vi "update.vi"(8 "error in (no error)":errorcluster, 11 "ScanHeadMH100729FPGA in":refnum<class "ScanHeadMH100729FPGA.lvclass">) -> (0 "error out":errorcluster, 3 "ScanHeadMH100729FPGA out":refnum<class "ScanHeadMH100729FPGA.lvclass">)   [LabVIEW 2010, in "ScanHeadMH100729FPGA.lvclass"]
uses:
  ScanHeadMH100729FPGA.lvclass
  Trajectory/GenericTrajectory/GenericTrajectory/GenericTrajectory.lvclass
  Trajectory/TrajectoryMG100122GenericFPGA/TrajectoryMG100122GenericFPGA/TrajectoryMG100122GenericFPGA.lvclass
  ScanHeadMH100729FPGA.lvclass/ScanHeadMH100729FPGA.ctl
  AnalogOut/GenericAnalogOut/GenericAnalogOut/GenericAnalogOut.lvclass
  common/classes/SpaceVector/SpaceVector/SpaceVector.lvclass
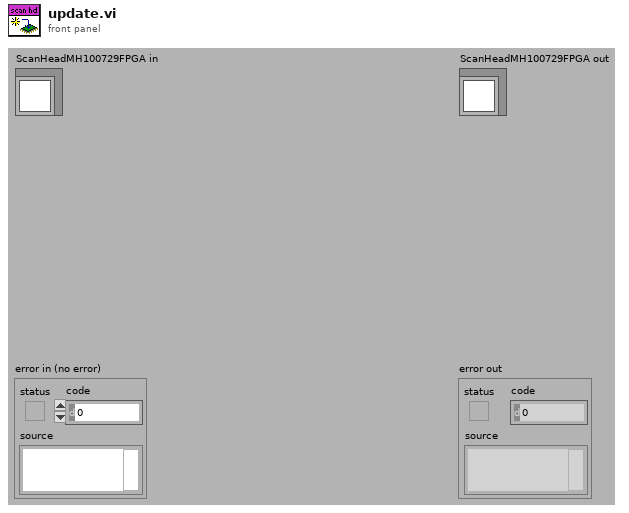
[diagram p1: front panel]
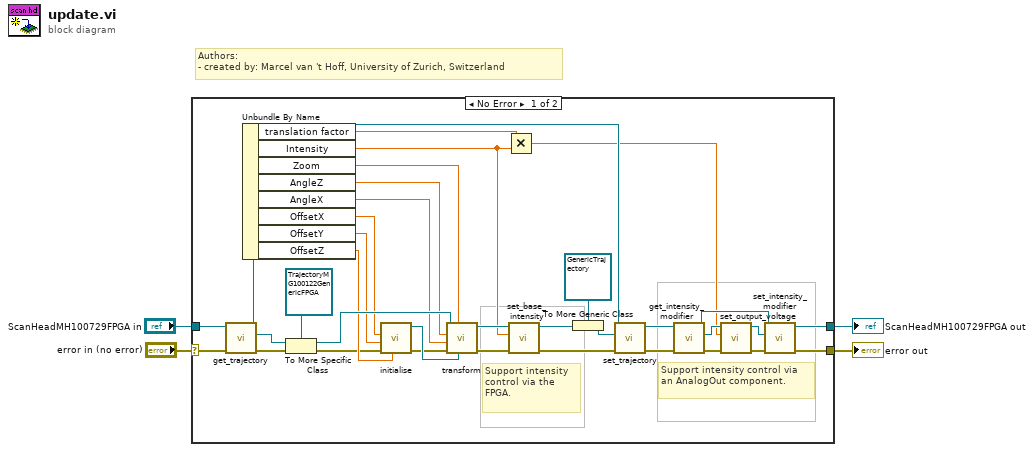
[diagram p0: block diagram]
diagram:
  # "Authors: \n- created by: Marcel van 't Hoff, University of Zurich, Switzerland"
  n1 = case shown="No Error" "error in (no error)" {
    selector: "error in (no error)" -> [w38 w40]
    tunnel: [w19 w40] -> w3
    tunnel: [w17 w39] -> w1
    tunnel: "ScanHeadMH100729FPGA in" -> [w37 w39]
    frame No Error {
      # "Support intensity control via the FPGA."
      # "Support intensity control via an AnalogOut component."
      n2 = call-dynamic "get_trajectory.vi"("error in (no error)"=w38, "GenericScanHead.lvclass in"=w37) -> ("error out"=w36:errorcluster, "trajectory"=w35:refnum<class "GenericTrajectory.lvclass">, "GenericScanHead.lvclass out"=w24:refnum<class "ScanHeadMH100729FPGA.lvclass">)  [unwired: 7 in]
      n3 = Unbundle By Name(w24) -> ("translation factor"=w12:dbl[unit], "Intensity"=w5:dbl, "Zoom"=w32:dbl, "AngleZ"=w31:dbl[unit], "AngleX"=w30:dbl[unit], "OffsetX"=w29:dbl[unit], "OffsetY"=w28:dbl[unit], "OffsetZ"=w27:dbl[unit])
      n4 = To More Specific Class(target class=refnum<class "TrajectoryMG100122GenericFPGA.lvclass"> refnum ("TrajectoryMG100122GenericFPGA.lvclass"), reference=w35, error in=w36) -> (specific class reference=w33:refnum<class "TrajectoryMG100122GenericFPGA.lvclass">, error out=w23:errorcluster)
      n5 = call "initialise.vi"("z"=w27, "error in (no error)"=w23, "y"=w28, "x"=w29) -> ("error out"=w22:errorcluster, "SpaceVector out"=w26:refnum<class "SpaceVector.lvclass">)  [unwired: 6 in]
      n6 = call-dynamic "transform.vi"("SpaceVector.lvclass"=w26, "zoom"=w32, "error in (no error)"=w22, "x angle (psi)"=w30, "z angle (phi)"=w31, "TrajectoryMG100122GenericFPGA in"=w33) -> ("error out"=w10:errorcluster, "TrajectoryMG100122GenericFPGA out"=w8:refnum<class "TrajectoryMG100122GenericFPGA.lvclass">)  [unwired: 4 in]
      n7 = Multiply(x=w12, y=w5) -> (x*y=w11:dbl[unit])
      n8 = call-dynamic "set_base_intensity.vi"("error in (no error)"=w10, "base intensity"=w5, "TrajectoryMG100122GenericFPGA in"=w8) -> ("error out"=w9:errorcluster, "TrajectoryMG100122GenericFPGA out"=w7:refnum<class "TrajectoryMG100122GenericFPGA.lvclass">)  [unwired: 7 in]
      n9 = To More Generic Class(target class=refnum<class "GenericTrajectory.lvclass"> refnum ("GenericTrajectory.lvclass"), reference=w7) -> (generic class reference=w6:refnum<class "GenericTrajectory.lvclass">)
      n10 = call-dynamic "set_trajectory.vi"("error in (no error)"=w9, "trajectory"=w6, "GenericScanHead.lvclass in"=w24) -> ("error out"=w18:errorcluster, "GenericScanHead.lvclass out"=w21:refnum<class "ScanHeadMH100729FPGA.lvclass">)  [unwired: 7 in]
      n11 = call-dynamic "get_intensity_modifier.vi"("error in (no error)"=w18, "ScanHeadMH100729FPGA in"=w21) -> ("error out"=w16:errorcluster, "intensity modifier"=w13:refnum<class "GenericAnalogOut.lvclass">, "ScanHeadMH100729FPGA out"=w20:refnum<class "ScanHeadMH100729FPGA.lvclass">)  [unwired: 7 in]
      n12 = call-dynamic "set_output_voltage.vi"("error in (no error)"=w16, "output value"=w11, "GenericAnalogOut in"=w13) -> ("error out"=w15:errorcluster, "GenericAnalogOut out"=w14:refnum<class "GenericAnalogOut.lvclass">)  [unwired: 7 in]
      n13 = call-dynamic "set_intensity_modifier.vi"("error in (no error)"=w15, "intensity modifier"=w14, "ScanHeadMH100729FPGA in"=w20) -> ("error out"=w19:errorcluster, "ScanHeadMH100729FPGA out"=w17:refnum<class "ScanHeadMH100729FPGA.lvclass">)  [unwired: 7 in]
    }
    frame Error {
    }
  }
  "error out" <- w3
  "ScanHeadMH100729FPGA out" <- w1
